vi "Decode.vi"(10 "ParamConfig":T1[](array[typedef]), 11 "Words In":u16[](array[numeric])) -> (3 "Parameters out":dbl[](array[numeric]))   [LabVIEW 2020]
uses:
  _typedefs/parameter_config_encoding_type.ctl
  _typedefs/parameter_config_type_type.ctl
  _typedefs/parameter_config_type.ctl
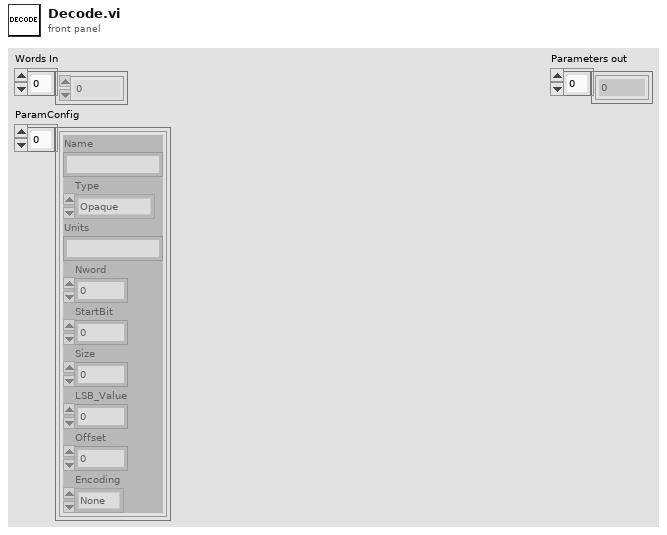
[diagram p1: front panel]
types:
  T1 = typedef "parameter_config_type.ctl" = cluster{"Name":string, "Type":T2, "Units":string, "Nword":i32, "StartBit":i32, "Size":i32, "LSB_Value":i32, "Offset":i32, "Encoding":T3}
  T2 = typedef "parameter_config_type_type.ctl" = enum16{"Opaque", "Enum", "Float", "Integer", "Bcd", "Bool"}
  T3 = typedef "parameter_config_encoding_type.ctl" = enum16{"None", "2-complement", "Unsigned"}
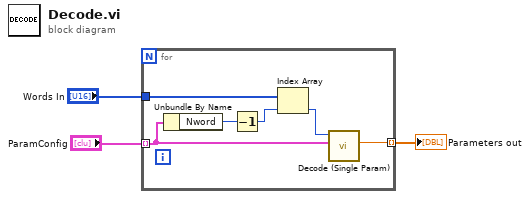
[diagram p0: block diagram]
diagram:
  n1 = for {
    tunnel: "Words In" -> [w9]
    tunnel: "ParamConfig" -> [w5] mode=indexing
    tunnel: [w4] -> w1 mode=indexing
    n2 = Unbundle By Name(w5) -> ("Nword"=w8:i32)
    n3 = Decrement(x=w8) -> (x-1=w7:i32)
    n4 = Index Array(array=w9, index=w7) -> (element=w6:u16)
    n5 = call "Decode (Single Param).vi"("parameter configuration"=w5, "Word in"=w6) -> ("Parameter Value out"=w4:dbl)  [unwired: 8 in, 1 out]
  }
  "Parameters out" <- w1
